vi "Fetch Multi Eval Meas IEM Margin Results.vi"(8 "error in (no error)":errorcluster, 9 "Result Type (Current)":i32(ring) items=["Current", "Average", "Extreme", "Standard Deviation"], 10 "Instance (1)":T2=1, 11 "VISA resource name":refnum<visa-resource-name>) -> (0 "error out":errorcluster, 1 "Margin Results":T1 {"Carrier Leakage" format="%^.3e"; "IQ Image" format="%^.3e"; "General" format="%^.3e"; "Out Of Tolerance" format="%^.3e"}, 2 "Reliability":i32, 3 "VISA resource name out":refnum<visa-resource-name>)   [LabVIEW 2015, in "Rohde&Schwarz CMXP NR FR2 Measurement.lvlib"]
doc: "Returns the multi eval measurement IEM limit line margin results.\n\nAttributes:\nRSCMXPNRFR2M_ATTR_FETCH_MULTI_EVAL_MEASUREMENT_IEM_MARGIN_AVERAGE_RESULTS\nRSCMXPNRFR2M_ATTR_FETCH_MULTI_EVAL_MEASUREMENT_IEM_MARGIN_CURRENT_RESULTS\nRSCMXPNRFR2M_ATTR_FETCH_MULTI_EVAL_MEASUREMENT_IEM_MARGIN_EXTREME_RESULTS\nRSCMXPNRFR2M_ATTR_FETCH_MULTI_EVAL_MEASUREMENT_IEM_MARGIN_STANDARD_DEVIATION_RESULTS\n\nRemote-control commands:\nFETCh:NRMMw:MEAS<i>:MEValuation:IEMission:MARGin:AVERage?\nFETCh:NRMMw:MEAS<i>:MEValuation:IEMission:MARGin:CURRent?\nFETCh:NRMMw:MEAS<i>:MEValuation:IEMission:MARGin:EXTReme?\nFETCh:NRMMw:MEAS<i>:MEValuation:IEMission:MARGin:SDEViation?"
uses:
  <instrlib>/Rohde&Schwarz CMXP NR FR2 Measurement/Rohde&Schwarz CMXP NR FR2 Measurement.lvlib
  <instrlib>/Rohde&Schwarz CMXP NR FR2 Measurement/Private/_Instance.ctl
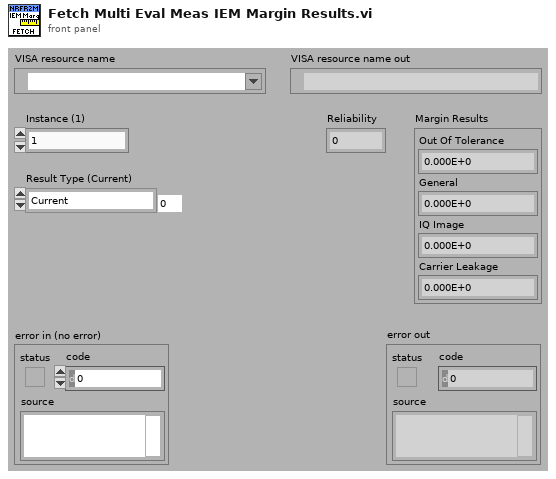
[diagram p1: front panel]
types:
  T1 = cluster{"Out Of Tolerance":dbl, "General":dbl, "IQ Image":dbl, "Carrier Leakage":dbl}
  T2 = typedef "Rohde&Schwarz CMXP NR FR2 Measurement.lvlib/_Instance.ctl" = i32
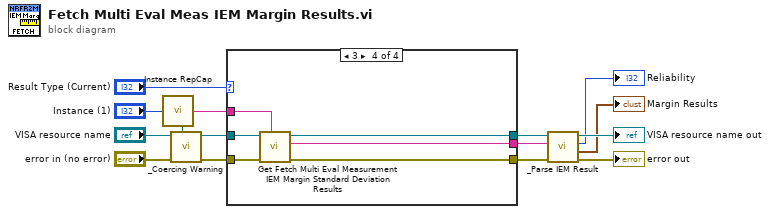
[diagram p0: block diagram]
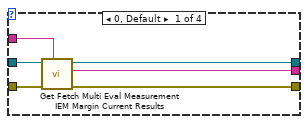
[diagram p2: hidden frame]
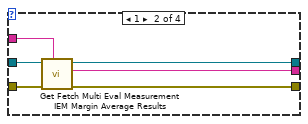
[diagram p3: hidden frame]
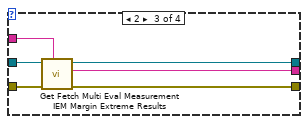
[diagram p4: hidden frame]
diagram:
  n1 = call <instrlib>:"Instance RepCap.vi"("Instance In"="Instance (1)") -> ("In Range?"=w6:bool, "RepCap Identifier Out"=w14:string)  [unwired: 1 in]
  n2 = call <instrlib>:"_Coercing Warning.vi"("In Range?"=w6, "error in (no error)"="error in (no error)", "VISA resource name"="VISA resource name") -> ("error out"=w4:errorcluster, "VISA resource name out"=w5:refnum<visa-resource-name>)  [unwired: 7 in]
  n3 = case shown="3" "Result Type (Current)" {
    tunnel: w4 -> [w20 w27 w33 w39]
    tunnel: w5 -> [w21 w26 w32 w38]
    tunnel: [w19 w25 w31 w37] -> w13
    tunnel: [w18 w24 w30 w36] -> w12
    tunnel: [w17 w23 w29 w35] -> w9
    tunnel: w14 -> [w16 w22 w28 w34]
    frame 0, Default {
      n4 = call "Get Fetch Multi Eval Measurement IEM Margin Current Results"("Repeated Capabilities"=w16, "error in (no error)"=w20, "instrument handle"=w21) -> ("error out"=w19:errorcluster, "Fetch Multi Eval Measurement IEM Margin Current Results"=w17:string, "instrument handle out"=w18:refnum<visa-resource-name>)  [unwired: 6 in]
    }
    frame 1 {
      n5 = call "Get Fetch Multi Eval Measurement IEM Margin Average Results"("Repeated Capabilities"=w22, "error in (no error)"=w27, "instrument handle"=w26) -> ("error out"=w25:errorcluster, "Fetch Multi Eval Measurement IEM Margin Average Results"=w23:string, "instrument handle out"=w24:refnum<visa-resource-name>)  [unwired: 6 in]
    }
    frame 2 {
      n6 = call "Get Fetch Multi Eval Measurement IEM Margin Extreme Results"("Repeated Capabilities"=w28, "error in (no error)"=w33, "instrument handle"=w32) -> ("error out"=w31:errorcluster, "Fetch Multi Eval Measurement IEM Margin Extreme Results"=w29:string, "instrument handle out"=w30:refnum<visa-resource-name>)  [unwired: 6 in]
    }
    frame 3 {
      n7 = call "Get Fetch Multi Eval Measurement IEM Margin Standard Deviation Results"("Repeated Capabilities"=w34, "error in (no error)"=w39, "instrument handle"=w38) -> ("error out"=w37:errorcluster, "Fetch Multi Eval Measurement IEM Margin Standard Deviation Results"=w35:string, "instrument handle out"=w36:refnum<visa-resource-name>)  [unwired: 6 in]
    }
  }
  n8 = call <instrlib>:"_Parse IEM Result.vi"("error in (no error)"=w13, "Input String"=w9, "VISA resource name"=w12) -> ("error out"=→"error out":errorcluster, "Result"=→"Margin Results":T1, "Reliability"=→"Reliability":i32, "VISA resource name out"=→"VISA resource name out":refnum<visa-resource-name>)  [unwired: 5 in]
